vi "Pop Out Error Message.vi"(7 "Pop Out Message":string, 11 "Error In":errorcluster) -> (3 "Error Out":errorcluster)   [LabVIEW 2022 SP3]
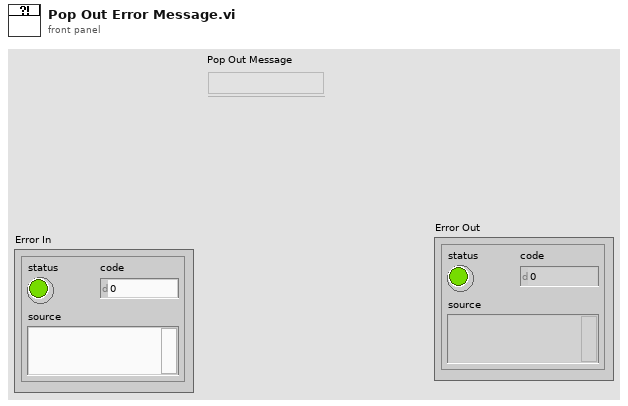
[diagram p1: front panel]
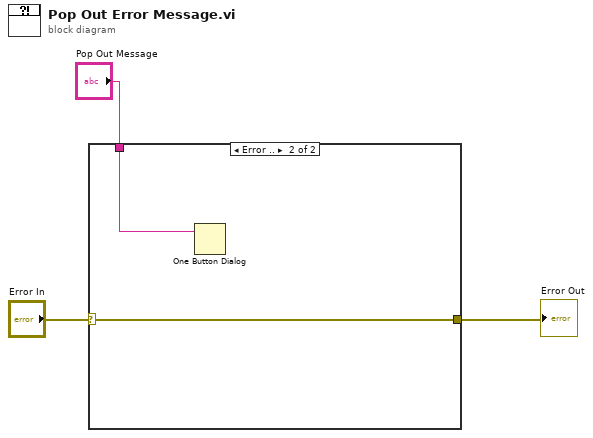
[diagram p0: block diagram]
diagram:
  n1 = case shown="Error .." "Error In" {
    selector: "Error In" -> [w4 w6]
    tunnel: [w4 w6] -> w2
    tunnel: "Pop Out Message" -> [_ w5]
    frame No Error {
    }
    frame Error {
      n2 = One Button Dialog(message=w5) -> ()  [unwired: 1 in, 1 out]
    }
  }
  "Error Out" <- w2
